vi "Impulse_Data_Processing.vi"() -> ()   [LabVIEW 2014]
uses:
  <vilib>/Simulation/Scripting/Companion Diagram/SimConfigNode/SimDog.xnode
  <vilib>/Simulation/Implementation/Shared/SIMSCR Execution Mode.ctl
  <vilib>/Simulation/Scripting/Companion Diagram/SimConfigNode/_simSolvers.ctl
  <vilib>/Simulation/Scripting/Companion Diagram/SimConfigNode/SimParams.ctl
  <vilib>/ptbypt/Signal Generation.llb/Gaussian White Noise PtByPt.vi
  <vilib>/ptbypt/NI_PtbyPt.lvlib
  <vilib>/Simulation/Implementation/XNodeFramework/SimXNode/SimX.xnode
  <vilib>/Simulation/SignalDisplay/Implementation/NILVSim Time Waveform.llb/SIM Time Waveform (scalar).vi
  <vilib>/Simulation/ContinuousLinear/Implementation/NILVSim Transfer Function.llb/SIM Transfer Function (SISO).vi
  <vilib>/Simulation/DataSources/Implementation/NILVSim Pulse Generator.llb/SIM Pulse Generator (scalar).vi
  <vilib>/Simulation/Implementation/Shared/SIM Bundle Sim Info.vi
  <vilib>/Simulation/Implementation/Shared/SIM Unbundle Sim Info.vi
  <vilib>/Simulation/Implementation/Shared/NILVSim_FinalizeModel.vi
  <vilib>/Simulation/Implementation/Shared/NILVSim_GetModelError.vi
  <vilib>/Simulation/Implementation/Shared/NILVSim_Initialize.vi
  <vilib>/Simulation/Utility/Implementation/NILVSim Get Time and IsAcceptedStep.vi
  <vilib>/Simulation/Implementation/Shared/NILVSim_Manager.vi
  <vilib>/Simulation/Implementation/Shared/NI_SIM_Implementation.lvlib
  <vilib>/Simulation/Implementation/Shared/NILVSIM_BeginStep.vi
  <vilib>/Simulation/Param Hierarchy/Typedefs/SIMPH Param Control Actions.ctl
  <vilib>/Simulation/Implementation/Shared/NILVSim_ParamChanged.vi
  <vilib>/Utility/error.llb/Clear Errors.vi
  <vilib>/Simulation/Implementation/Shared/SIMSH Read Queue.vi
  <vilib>/Simulation/ContinuousLinear/Implementation/NILVSim Transfer Function.llb/SIM Transfer Function Collector (SISO).vi
  <vilib>/Simulation/ContinuousLinear/Implementation/NILVSim Transfer Function.llb/SIM Transfer Function Distributor (SISO).vi
panel:
  out "size(s)":i32
  out "array":dbl[][](array[numeric])
  in  "file path (use dialog)":path=path "D:/Academic_Gaduate/Course/2016 Spring/2.131/Project/MyRIO/DAQ and Actuation DIO Stochastic Double Input 125kHz differential measurement and system ID with Bode Plot Analysis/04212016/RC/BinaryStochastic/042116_RC_Stochastic_3.csv"
  out "Phase spectrum":cluster{"f0":dbl, "df":dbl, "phase":dbl[]}(graph)={"f0"=0.0, "df"=20.115867396202123, "phase"=array[24856 elements]}
  out "Amplitude spectrum":cluster{"f0":dbl, "df":dbl, "magnitude":dbl[]}(graph)={"f0"=0.0, "df"=20.115867396202123, "magnitude"=array[24856 elements]}
  in  "Freq (Hz)":dbl=125000.0
  out "Output":waveform(i16)(graph)={"t0"=timestamp(0 s since 1904-01-01), "dt"=2e-06, "Y"=array[24857 elements]}
  out "Input":waveform(i16)(graph)={"t0"=timestamp(0 s since 1904-01-01), "dt"=2e-06, "Y"=array[24857 elements]}
  out "System ID":waveform(dbl)(graph)={"t0"=timestamp(0 s since 1904-01-01), "dt"=2e-06, "Y"=[]}
  in  "CS_R(ohm)":dbl=500000.0
  in  "INA R(ohm)":dbl=1000.0
  out "Waveform Chart":waveform(dbl)(graph)={"t0"=timestamp(0.01 s since 1904-01-01), "dt"=1.0, "Y"=[1.8810764409104788]}
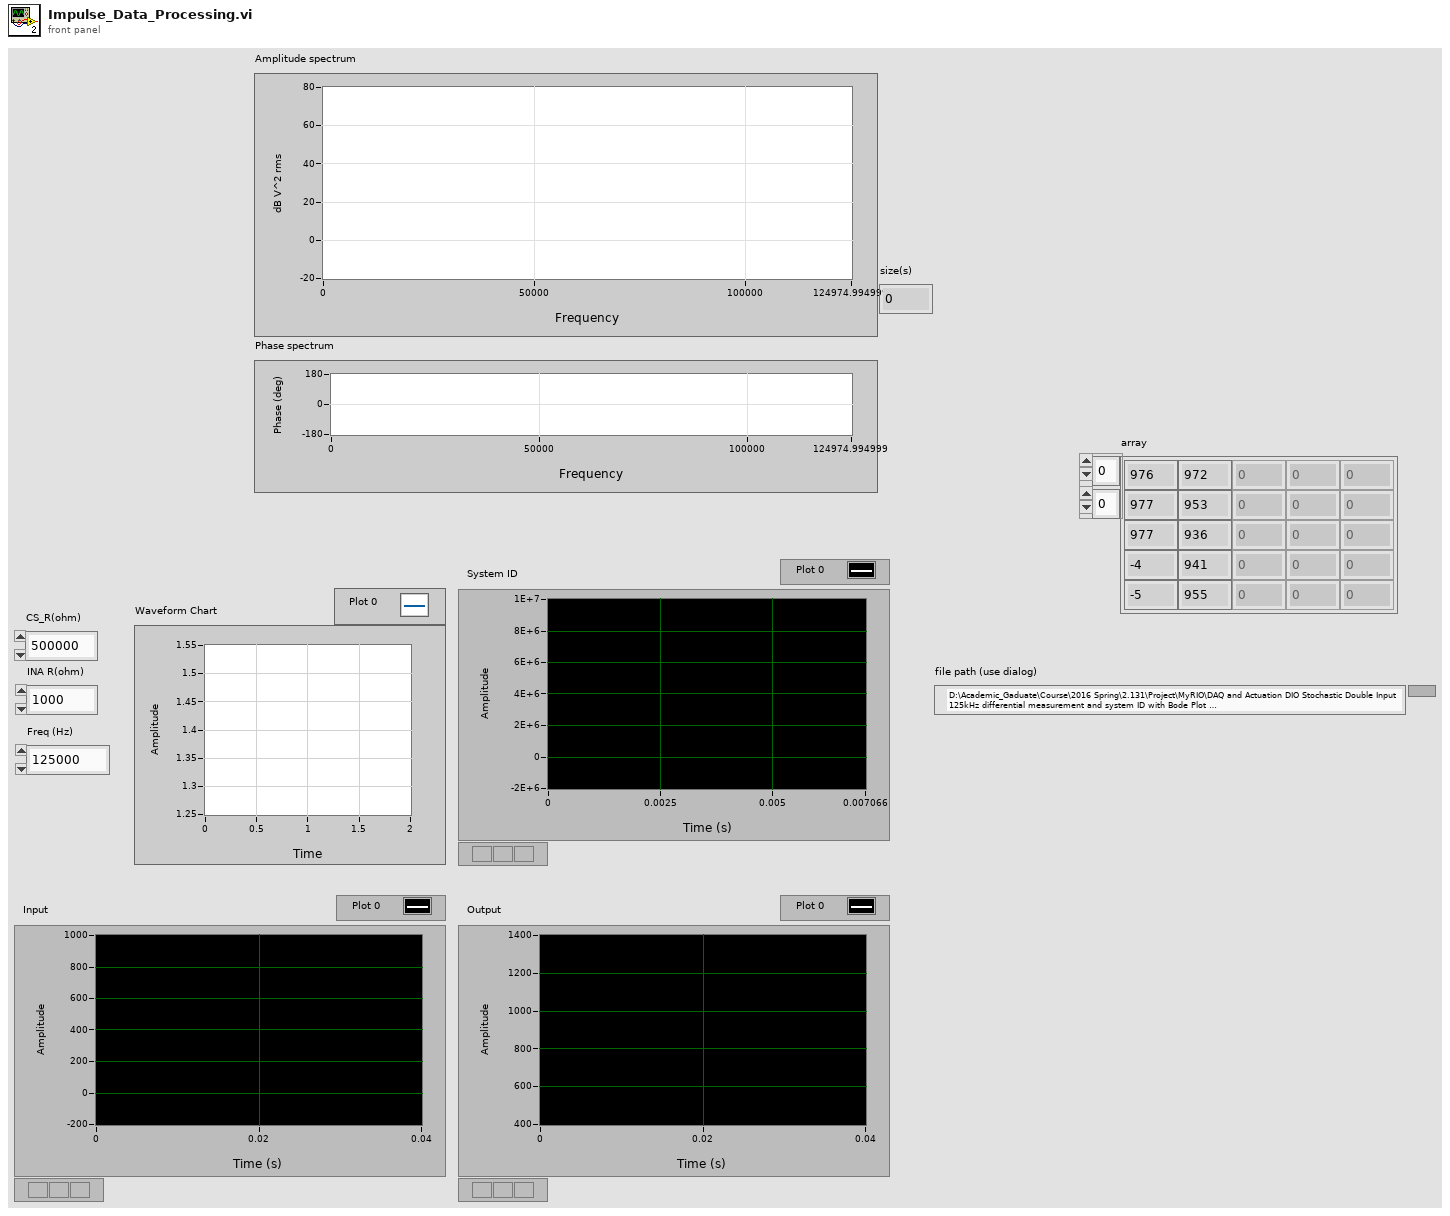
[diagram p1: front panel]
types:
  T1 = enum16{"open", "replace", "create", "open or create", "replace or create", "replace or create with confirmation"}
  T2 = typedef "SIMSCR Execution Mode.ctl" = enum16{"Simulate to Completion", "Single Time-Step Simulation (Fixed Step Only)"}
  T3 = typedef "SIMPH Param Control Actions.ctl" = enum16{"get params", "set params"}
  T4 = typedef "SimParams.ctl" = cluster{"Initial Time (s)":dbl, "Final Time (s)":dbl, "Step Size (s)":dbl, "ODE Solver":T5, "Minimum Step Size (s)":dbl, "Maximum Step Size (s)":dbl, "Relative Tolerance":dbl, "Absolute Tolerance":dbl, "Software Timing":bool, "Initial Step Size (s)":dbl, "Automatic Fixed Step Size?":bool, "Automatic Discrete Step Size?":bool, "Discrete Step Size (s)":dbl, "Calculate using Time Step":bool, "Solver Wired?":bool, "Prev.Frm.Expected End":u64, "Prev.Frm.Actual End":u64, "Prev.Frm.Finished Late?":bool, "Prev.Iter.Expected End":u64, "Prev.Iter.Actual End":u64, "Prev.Iter.Finished Late?":bool, "Expected Iteration Start":u64, "Actual Iteration Start":u64, "Expected Frame Start":u64, "Actual Frame Start":u64, "Source Name":string, "Name":string, "Period":i64, "Deadline":i64, "Offset":i64, "Start":i64, "Priority":i32, "Timeout":i32, "Processor":i32, "Mode":enum32{"No Change", "Process missed periods, maintain original phase", "Discard missed periods, maintain original phase", "Process missed periods, ignore original phase", "Discard missed periods, ignore original phase"}, "Wakeup reason":enum32{"Normal", "Aborted", "Asynchronous wakeup", "Timing source error", "Timed loop error", "Timeout"}, "Error":errorcluster, "Source Type":string, "Secondary Source Type":string, "Global End Time":u64, "Global Start Time":u64, "Full Solver Reset":bool, "Execution Mode":T2, "Nan/Inf Check":bool, "Custom Solver Library":string, "Solver Is Variable":bool, "custom solver name":string, "Signal Collection Decimation":u32}
  T5 = typedef "_simSolvers.ctl" = enum16{"Runge-Kutta 1 (Euler)", "Runge-Kutta 2", "Runge-Kutta 3", "Runge-Kutta 4", "Runge-Kutta 23 (variable)", "Runge-Kutta 45 (variable)", "BDF (variable)", "Adams-Moulton (variable)", "Rosenbrock (variable)", "Discrete States Only", "SDIRK 4 (variable)", "Radau 5 (variable)", "Radau 9 (variable)", "Radau 13 (variable)", "Radau [Variable Order] (variable)", "Gear's Method (variable)", "Linearizer", "State Query", "Trim Eval", "Custom Solver"}
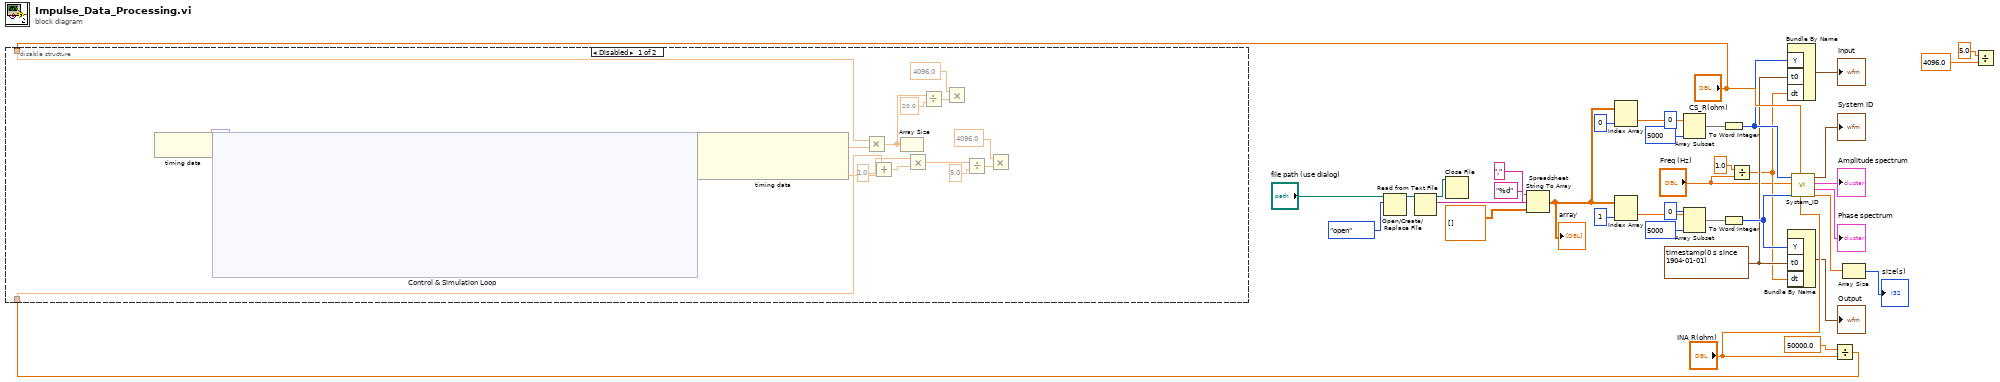
[diagram p0: block diagram]
diagram:
  (unwired) 0 ("length")
  w27 = timestamp(0 s since 1904-01-01) ("t0")
  n1 = Open/Create/Replace File(file path (use dialog)="file path (use dialog)", operation (0:open)=T1."open") -> (refnum out=w19:refnum<file>)  [unwired: 4 in, 2 out]
  n2 = Read from Text File(file (use dialog)=w19) -> (refnum out=w14:refnum<file>, text=w17:string)  [unwired: 3 in, 2 out]
  n3 = Close File(refnum=w14) -> ()  [unwired: 1 in, 2 out]
  n4 = Spreadsheet String To Array(delimiter (Tab)=",", format string="%d", spreadsheet string=w17, array type (2D Dbl)=dbl[][] []) -> (array=w10:dbl[][])
  "array" <- w10
  n5 = Index Array(array=w10, index (col)=0 ("disabled index (col)")) -> (element=w7:dbl[])  [unwired: 1 in]
  n6 = Index Array(array=w10, index (col)=1 ("disabled index (col)")) -> (element=w3:dbl[])  [unwired: 1 in]
  n7 = Array Subset(array=w7, length=5000) -> (w6:dbl[])  [unwired: 1 in]
  n8 = Array Subset(array=w3, index=0, length=5000) -> (w2:dbl[])
  n9 = To Word Integer(number=w6) -> (16bit integer=w31:i16[])
  n10 = To Word Integer(number=w2) -> (16bit integer=w28:i16[])
  n11 = Divide(x=1.0, y="Freq (Hz)") -> (x/y=w26:dbl)
  n12 = Bundle By Name("Y"=w31, "t0"=w27, "dt"=w26) -> (→"Input":waveform(i16))  [unwired: 1 in]
  n13 = Bundle By Name("Y"=w28, "t0"=w27, "dt"=w26) -> (→"Output":waveform(i16))  [unwired: 1 in]
  n14 = call "System_ID.vi"("INA Resistance (ohm)"="INA R(ohm)", "Current Source Resistance (ohm)"="CS_R(ohm)", "Input Y"=w28, "Sample_Frequency (Hz)"="Freq (Hz)", "Input X"=w31) -> ("x*y"=w32:dbl[], "Phase spectrum"=→"Phase spectrum":cluster{"f0":dbl, "df":dbl, "phase":dbl[]}, "Amplitude spectrum"=→"Amplitude spectrum":cluster{"f0":dbl, "df":dbl, "magnitude":dbl[]}, "Actuation Graph"=→"System ID":waveform(dbl))  [unwired: 3 in]
  n15 = Divide(x=50000.0, y="INA R(ohm)") -> (x/y=w36:dbl)
  n16 = disable-structure shown="Disabled" {
    disable-tunnel: w36 -> [w43 _]
    disable-tunnel: "CS_R(ohm)" -> [w40 _]
    frame Disabled {
      n17 = node-c288() -> (w53:variant)  [unwired: 1 in]
      n18 = node-c254 "Control & Simulation Loop"(w53) -> (w52:variant)
      n19 = node-c288(w52) -> (w39:dbl[], w41:dbl[])  [unwired: 1 out]
      n20 = Multiply(x=w40, y=w39) -> (x*y=w38:dbl[])
      n21 = Add(x=w43, y=1.0 ("x")) -> (x+y=w42:dbl)
      n22 = Array Size(array=w38) -> ()  [unwired: 1 out]
      n23 = Multiply(x=w41, y=w42) -> (x*y=w48:dbl[])
      n24 = Divide(x=w38, y=20.0 ("f")) -> (x/y=w50:dbl[])
      n25 = Multiply(x=4096.0 ("f"), y=w50) -> ()  [unwired: 1 out]
      n26 = Divide(x=w48, y=5.0 ("f")) -> (x/y=w46:dbl[])
      n27 = Multiply(x=4096.0 ("f"), y=w46) -> ()  [unwired: 1 out]
    }
    frame Enabled {
    }
  }
  n28 = Array Size(array=w32) -> (size(s)=→"size(s)":i32)
  n29 = Divide(x=5.0, y=4096.0) -> ()  [unwired: 1 out]
